vi "GUI_Camera_no_superGUI.vi"() -> ()   [LabVIEW 2013]
uses:
  Shared/GUI_Template/GUI_master/tcp_new_data_event.ctl
  Shared/GUI_Template/GUI_master/tcp new data cluster.ctl
panel:
  out "Image 2":T1(plugin-control)
  out "Image":T1(plugin-control)
  in  "stop":bool
  in  "GUIdevice 1":string="PL2-AndorCam"
  out "tcp data event":T2
  out "error IO 2":errorcluster
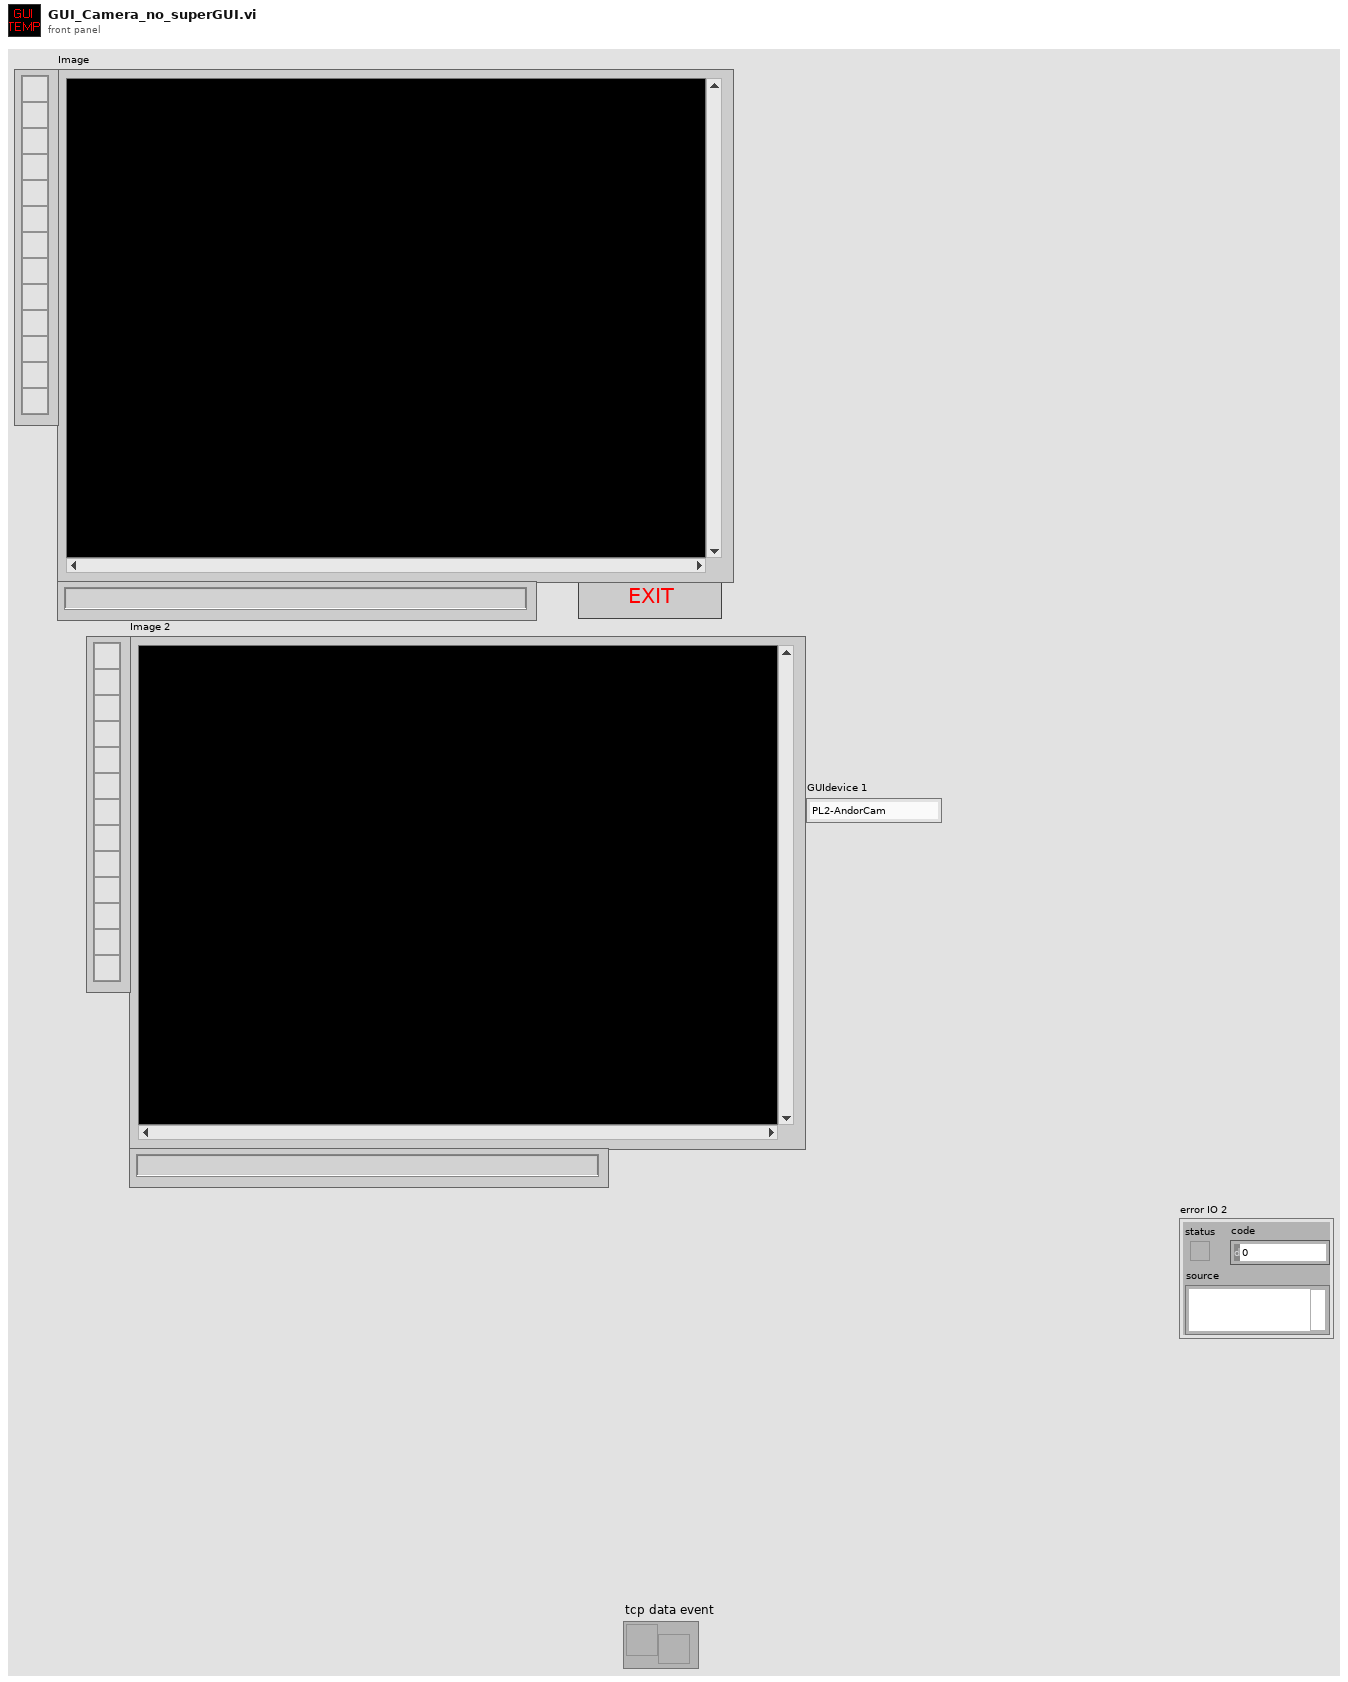
[diagram p1: front panel]
types:
  T1 = typedef "IMAQ Image.ctl" = refnum<image>
  T2 = typedef "tcp_new_data_event.ctl" = refnum<user-event>
  T3 = typedef "tcp new data cluster.ctl" = cluster{"EventEnum":enum16{"new data", "connection status update"}, "Device name":string}
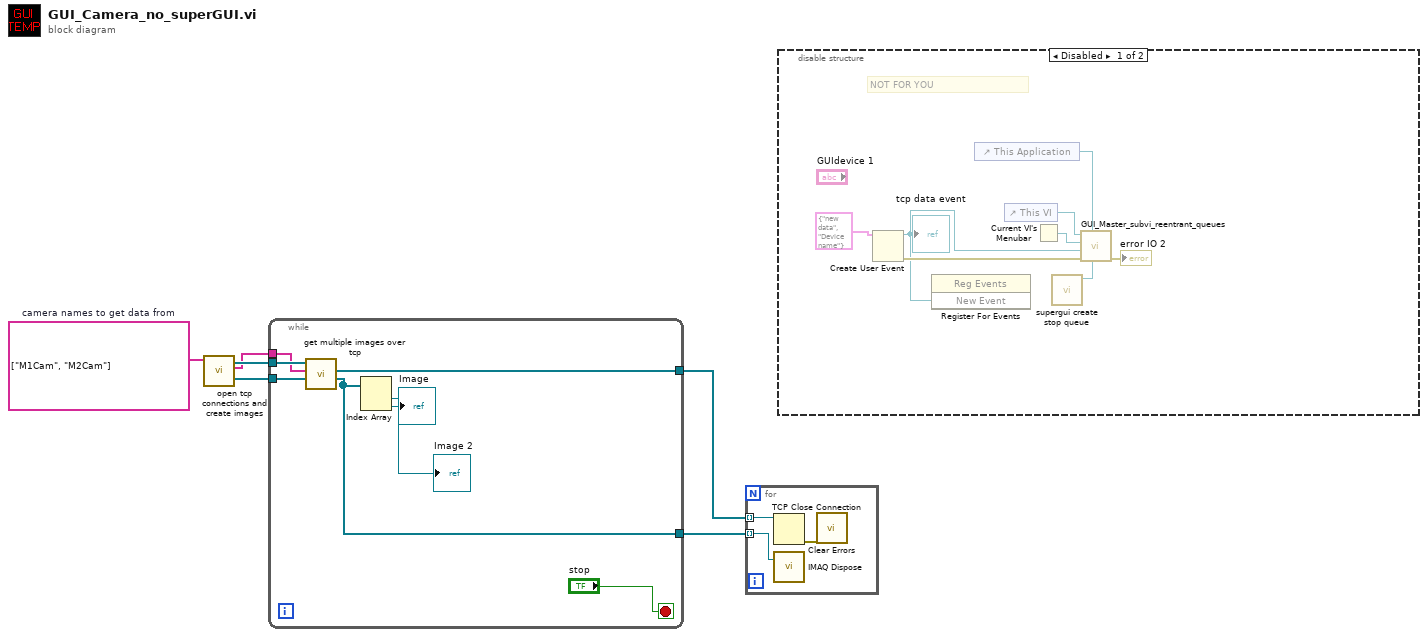
[diagram p0: block diagram]
diagram:
  w6 = string[] ["M1Cam", "M2Cam"]  # camera names to get data from
  n1 = call "open tcp connections and create images.vi"("devices to get data from"=w6) -> ("images"=w4:T1[], "subscribe messages\nfor process vis"=w3:string[], "tcp connections"=w5:refnum<k5>[])  [unwired: 8 in]
  n2 = while {
    tunnel: w5 -> [w13]
    tunnel: w4 -> [w12]
    tunnel: w3 -> [w11]
    tunnel: [w8] -> w2
    tunnel: [w7] -> w1
    stop <- "stop" stop-if-true
    n3 = call "get multiple images over tcp.vi"("images In"=w12, "subscribeMessages"=w11, "TCP_Refs In"=w13) -> ("Images out"=w7:T1[], "TCP_Refs_out"=w8:refnum<k5>[])  [unwired: 4 in, 3 out]
    n4 = Index Array(array=w7) -> (element #1=→"Image":T1, element #2=→"Image 2":T1)  [unwired: 2 in]
  }
  n5 = for {
    tunnel: w2 -> [w17] mode=indexing
    tunnel: w1 -> [w16] mode=indexing
    n6 = TCP Close Connection(connection ID=w17) -> (error out=w15:errorcluster)  [unwired: 2 in, 1 out]
    n7 = call "IMAQ Dispose"("Image"=w16) -> ()  [unwired: 5 in, 1 out]
    n8 = call <vilib>:"Clear Errors.vi"("error in (no error)"=w15) -> ()  [unwired: 6 in, 1 out]
  }
  n9 = disable-structure shown="Disabled" {
    frame Disabled {
      # "NOT FOR YOU"
      n10 = Create User Event(user event datatype=T3 {"EventEnum"=enum."new data", "Device name"="Device name"} ("New Event")) -> (user event=w20:refnum<user-event>, error out=w21:errorcluster)  [unwired: 1 in]
      "tcp data event" <- w20
      n11 = register-events(w20) -> ()  [unwired: 2 in, 2 out]
      n12 = control-ref of="This Application"() -> (w19:refnum<vi>)
      n13 = control-ref of="This VI"() -> (w24:refnum<vi>)
      n14 = Current VI's Menubar() -> (w23:refnum<k9>)
      n15 = call "supergui create stop queue.vi"() -> ("STOP Queue out"=w18:refnum<queue>)  [unwired: 11 in]
      n16 = call "GUI_Master_subvi_reentrant_queues.vi"("STOP Queue in"=w18, "This Application"=w19, "error in (no error)"=w21, "tcp data event"=w20, "Caller menu reference"=w23, "Caller VI ref"=w24) -> ("error out"=→"error IO 2":errorcluster)  [unwired: 5 in]
    }
    frame Enabled {
    }
  }
